vi "Teleop.vi"(10 "Match Info":T13={"Autonomous Elapsed Seconds"=0.0, "TeleOp Elapsed Seconds"=0.0, "Disabled Elapsed Seconds"=0.0, "Visited Autonomous"=FALSE, "Visited TeleOp"=FALSE, "Visited Disabled"=FALSE, "Autonomous Settings"={"Autonomous Style"=enum."Independent", "VI Refnum"=refnum}}, 11 "Call Context":T14) -> ()   [LabVIEW 2014]
doc: "This VI is called for each TeleOp packet received from the DS where the robot is not disabled. It is often used to read from the joysticks and update I/O or to update setpoints for timed control loops. It should complete and return within 20 milliseconds or it may miss DS packets."
uses:
  <vilib>/Rock Robotics/WPI/DriverStation/WPI_DriverStationDerivedRobotMode.ctl
  <vilib>/Rock Robotics/WPI/DriverStation/WPI_DriverStationMatch Info.ctl
  <vilib>/Rock Robotics/WPI/Joystick/WPI_JoystickDevRef.ctl
  <vilib>/Rock Robotics/WPI/Joystick/WPI_JoystickDeviceEnum.ctl
  <vilib>/Rock Robotics/WPI/RobotDrive/WPI_RobotDriveDevRef.ctl
  <vilib>/Rock Robotics/WPI/MotorControl/WPI_MotorControlDeviceRef.ctl
  <vilib>/Rock Robotics/WPI/MotorControl/WPI_MotorControlType.ctl
  <vilib>/Rock Robotics/SystemInterfaces/Typedef/FPGA_TypedefDigitalModule.ctl
  <vilib>/Rock Robotics/SystemInterfaces/DIO/FPGA_DIOPWMChannel.ctl
  <vilib>/Rock Robotics/WPI/PWM/WPI_PWMDeadband.ctl
  <vilib>/Rock Robotics/WPI/CAN/Jaguar/SubVIs/WPI_CANJaguar_ControlMode.ctl
  <vilib>/Rock Robotics/WPI/CAN/TalonSRX/WPI_CANTalonSRX_APIControlMode.ctl
  <vilib>/Rock Robotics/WPI/PWM/WPI_PWMTransform_ConPane.ctl
  <vilib>/Rock Robotics/WPI/Solenoid/WPI_SolenoidValue.ctl
  <vilib>/Rock Robotics/Network Tables/SD Read Boolean.vi
  <vilib>/Rock Robotics/Network Tables/SD Read Number.vi
  <vilib>/Rock Robotics/WPI/Joystick/WPI_JoystickGetSetRefNum.vi
  <vilib>/Rock Robotics/Network Tables/SD Read Boolean Array.vi
  <vilib>/Rock Robotics/WPI/RobotDrive/WPI_RobotDriveGetSetRefNum.vi
  <vilib>/Rock Robotics/Network Tables/SD Write Numeric Array.vi
  Robot Global Data.vi
  <vilib>/Rock Robotics/WPI/Solenoid/WPI_SolenoidSetEnum.vi
  <vilib>/Rock Robotics/Network Tables/SD Write Boolean Array.vi
  <vilib>/Rock Robotics/WPI/RobotDrive/WPI_RobotDriveMecanumDrive_Cartesian.vi
panel:
  out "Mecanum_Motors":T1={"DevStatus"={"status"=FALSE, "code"=0, "source"=""}, "Motors[]"=[], "Square Inputs"=FALSE, "Max Output"=1.0}
  out "Numeric":dbl
  out "Boolean Array":bool[](array[boolean])
  in  "Radio Buttons":enum32{"Radio Selection 1", "Radio Selection 2"}(radio)
  out "Joystick_1":T11={"Device"=enum."USB 1"}
  out "Joystick_0":T11={"Device"=enum."USB 1"}
  out "Sample Slider 0":dbl(slide) scale=0.0..5.0
  out "Sample Boolean 1":bool
  out "Sample Boolean 0":bool
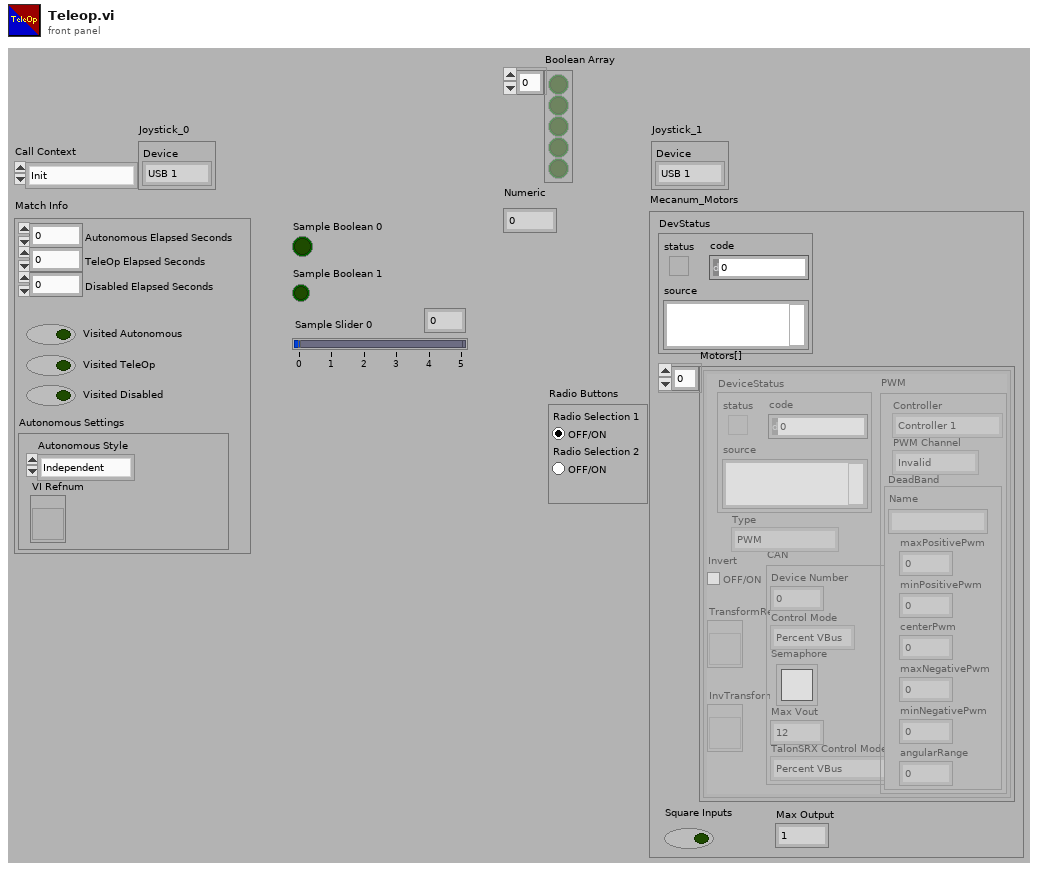
[diagram p1: front panel]
types:
  T1 = typedef "WPI_RobotDriveDevRef.ctl" = cluster{"DevStatus":errorcluster, "Motors[]":T2[], "Square Inputs":bool, "Max Output":dbl}
  T2 = typedef "WPI_MotorControlDeviceRef.ctl" = cluster{"DeviceStatus":errorcluster, "Type":T3, "PWM":cluster{"Controller":T4, "PWM Channel":T5, "DeadBand":T6}, "CAN":cluster{"Device Number":u8, "Control Mode":T7, "Semaphore":T8, "Max Vout":dbl, "TalonSRX Control Mode":T9}, "Invert":bool, "TransformRef":T10, "InvTransformRef":T10}
  T3 = typedef "WPI_MotorControlType.ctl" = enum16{"PWM", "CAN", "CANTalonSRX"}
  T4 = typedef "FPGA_TypedefDigitalModule.ctl" = enum16{"Controller 1"}
  T5 = typedef "FPGA_DIOPWMChannel.ctl" = enum8{"PWM 0", "PWM 1", "PWM 2", "PWM 3", "PWM 4", "PWM 5", "PWM 6", "PWM 7", "PWM 8", "PWM 9", "PWM MXP 0", "PWM MXP 1", "PWM MXP 2", "PWM MXP 3", "PWM MXP 4", "PWM MXP 5", "PWM MXP 6", "PWM MXP 7", "PWM MXP 8", "PWM MXP 9", "Invalid"}
  T6 = typedef "WPI_PWMDeadband.ctl" = cluster{"Name":string, "maxPositivePwm":i32, "minPositivePwm":i32, "centerPwm":i32, "maxNegativePwm":i32, "minNegativePwm":i32, "angularRange":u16}
  T7 = typedef "WPI_CANJaguar_ControlMode.ctl" = enum8{"Percent VBus", "Current", "Speed", "Position", "Voltage"}
  T8 = typedef "Semaphore RefNum" = refnum<k1>
  T9 = typedef "WPI_CANTalonSRX_APIControlMode.ctl" = enum8{"Percent VBus", "Speed", "Position", "Slave", "Unchanged / Invalid"}
  T10 = typedef "WPI_PWMTransform_ConPane.ctl" = refnum<vi>
  T11 = typedef "WPI_JoystickDevRef.ctl" = cluster{"Device":T12}
  T12 = typedef "WPI_JoystickDeviceEnum.ctl" = enum16{"USB 0", "USB 1", "USB 2", "USB 3", "USB 4", "USB 5"}
  T13 = typedef "WPI_DriverStationMatch Info.ctl" = cluster{"Autonomous Elapsed Seconds":dbl, "TeleOp Elapsed Seconds":dbl, "Disabled Elapsed Seconds":dbl, "Visited Autonomous":bool, "Visited TeleOp":bool, "Visited Disabled":bool, "Autonomous Settings":cluster{"Autonomous Style":enum16{"Iterative", "Independent"}, "VI Refnum":refnum<vi>}}
  T14 = typedef "WPI_DriverStationDerivedRobotMode.ctl" = enum16{"Init", "Execute", "Stop"}
  T15 = typedef "WPI_SolenoidValue.ctl" = enum16{"Off", "On", "Forward", "Reverse"}
  T16 = typedef "WPI_SolenoidDevRef.ctl" = cluster{"DevStatus":errorcluster, "Pneumatics Control Module":u8, "Forward Solenoid Channel":T17, "Reverse Solenoid Channel":T17}
  T17 = typedef "WPI_SolenoidChannel.ctl" = enum8{"Solenoid 0", "Solenoid 1", "Solenoid 2", "Solenoid 3", "Solenoid 4", "Solenoid 5", "Solenoid 6", "Solenoid 7", "Invalid"}
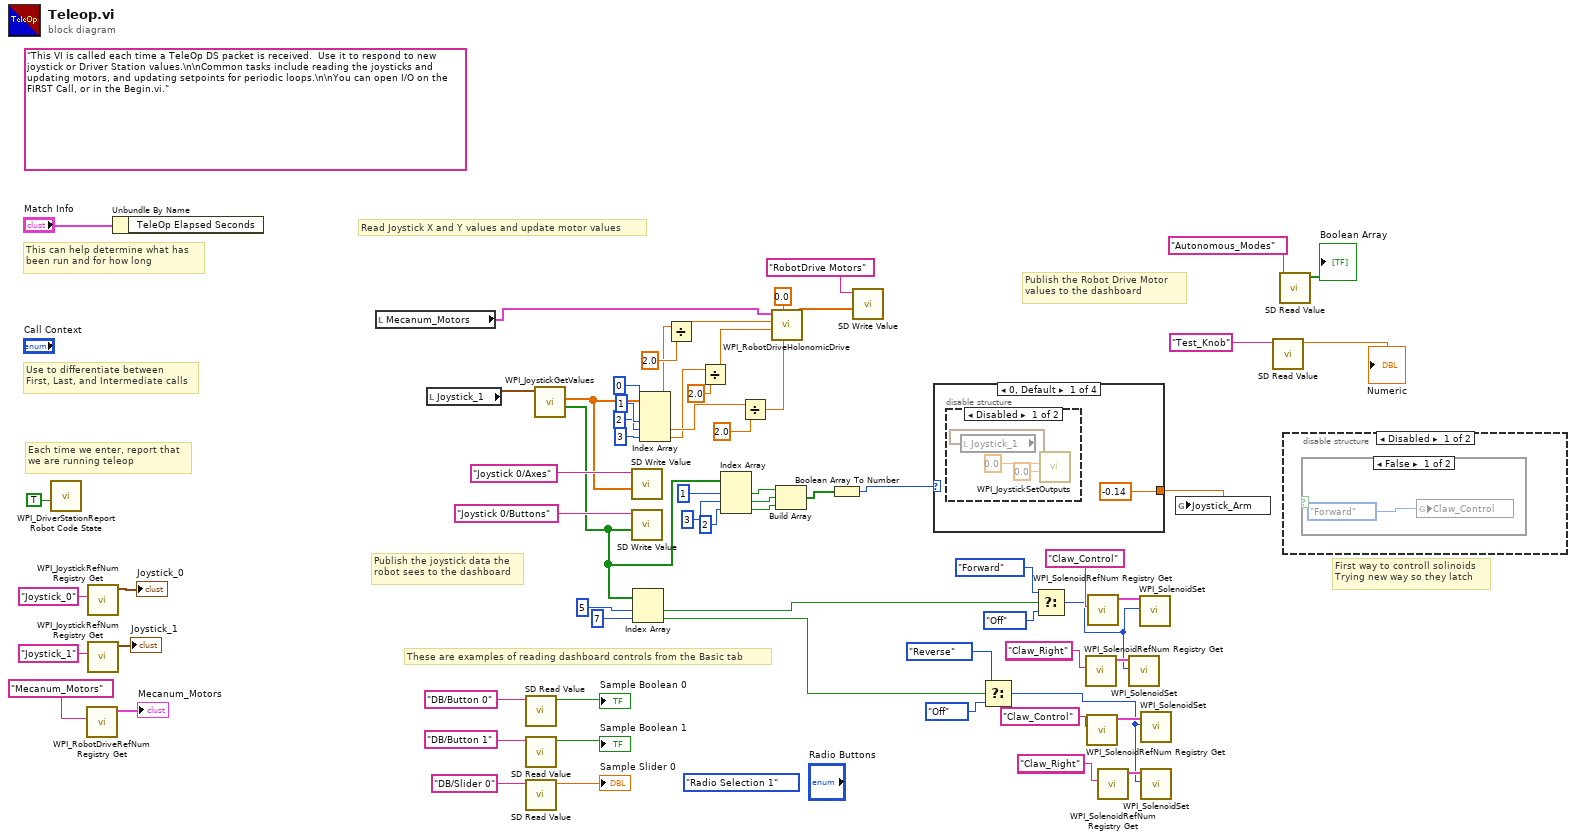
[diagram p0: block diagram]
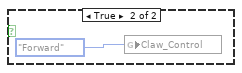
[diagram p2: hidden frame]
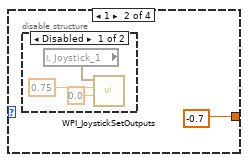
[diagram p5: hidden frame]
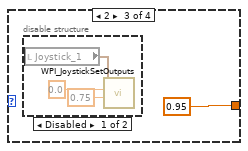
[diagram p7: hidden frame]
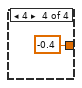
[diagram p9: hidden frame]
diagram:
  (unwired) "Claw_Right" ("refnum name")
  (unwired) "Claw_Right" ("refnum name")
  (unwired) enum32{"Radio Selection 1", "Radio Selection 2"}."Radio Selection 1" ("Radio Buttons")
  (unwired) "This VI is called each time a TeleOp DS packet is received.  Use it to respond to new joystick or Driver Station values.\n\nCommon tasks include reading the joysticks and updating motors, and updating setpoints for periodic loops.\n\nYou can open I/O on the FIRST Call, or in the Begin.vi."
  # "First way to controll solinoids\nTrying new way so they latch"
  # "These are examples of reading dashboard controls from the Basic tab"
  # "Publish the Robot Drive Motor\nvalues to the dashboard"
  # "Publish the joystick data the\nrobot sees to the dashboard"
  # "Each time we enter, report that\nwe are running teleop"
  # "Use to differentiate between\nFirst, Last, and Intermediate calls"
  # "This can help determine what has\nbeen run and for how long"
  # "Read Joystick X and Y values and update motor values"
  n1 = call <vilib>:"WPI_DriverStationReport Robot Code State.vi"("TeleOp"=TRUE ("Autonomous")) -> ()  [unwired: 10 in, 1 out]
  n2 = call <vilib>:"WPI_RobotDriveRefNum Registry Get.vi"("refnum name"="Mecanum_Motors") -> ("RobotDriveDevRef"=→"Mecanum_Motors":T1)  [unwired: 1 in, 9 out]
  n3 = call <vilib>:"WPI_JoystickRefNum Registry Get.vi"("refnum name"="Joystick_0") -> ("JoystickDevRef"=→"Joystick_0":T11)  [unwired: 9 in, 1 out]
  n4 = call <vilib>:"WPI_JoystickRefNum Registry Get.vi"("refnum name"="Joystick_1") -> ("JoystickDevRef"=→"Joystick_1":T11)  [unwired: 9 in, 1 out]
  n5 = Unbundle By Name("Match Info") -> ()  [unwired: 1 out]
  n6 = local read "Mecanum_Motors"() -> (w36:T1)
  n7 = local read "Joystick_1"() -> (w39:T11)
  n8 = call-poly <vilib>:"SD Read Value.vi"("Name"="DB/Button 0" ("refnum name")) -> ("Boolean"=→"Sample Boolean 0":bool)  [unwired: 8 in, 2 out]
  n9 = call-poly <vilib>:"SD Read Value.vi"("Name"="DB/Button 1" ("refnum name")) -> ("Boolean"=→"Sample Boolean 1":bool)  [unwired: 8 in, 2 out]
  n10 = call-poly <vilib>:"SD Read Value.vi"("Name"="DB/Slider 0" ("refnum name")) -> ("Numeric"=→"Sample Slider 0":dbl)  [unwired: 8 in, 2 out]
  n11 = call <vilib>:"WPI_JoystickGetValues.vi"("JoystickDevRef"=w39) -> ("Buttons"=w35:bool[], "Axes"=w51:dbl[])  [unwired: 6 in, 3 out]
  n12 = call-poly <vilib>:"SD Write Value.vi"("Numeric Array"=w51, "Name"="Joystick 0/Axes") -> ()  [unwired: 8 in, 2 out]
  n13 = call-poly <vilib>:"SD Write Value.vi"("Boolean Array"=w35, "Name"="Joystick 0/Buttons") -> ()  [unwired: 8 in, 2 out]
  n14 = Index Array(array=w35, index #1=5 ("index"), index #2=7 ("index")) -> (element #1=w27:bool, element #2=w16:bool)
  n15 = Index Array(array=w51, index #1=0, index #2=1, index #3=2 ("index"), index #4=3 ("index")) -> (element #1=w8:dbl, element #3=w13:dbl, element #4=w10:dbl)  [unwired: 1 out]
  n16 = Divide(x=w8, y=2.0) -> (x/y=w7:dbl)
  n17 = Divide(x=w10, y=2.0) -> (x/y=w9:dbl)
  n18 = Index Array(array=w35, index #1=1, index #2=3, index #3=2 ("index")) -> (element #1=w32:bool, element #2=w31:bool, element #3=w17:bool)
  n19 = Divide(x=w13, y=2.0) -> (x/y=w15:dbl)
  n20 = call-poly <vilib>:"WPI_RobotDriveHolonomicDrive.vi"("Rotation"=w15, "Gyro Angle"=0.0, "Y"=w9, "X"=w7, "RobotDriveDevRef"=w36) -> ("Motor Values"=w58:dbl[])  [unwired: 4 in, 2 out]
  n21 = Build Array(w32, w31, w17) -> (w30:bool[])
  n22 = Boolean Array To Number(Boolean array=w30) -> (number=w29:u32)
  n23 = call-poly <vilib>:"SD Write Value.vi"("Numeric Array"=w58, "Name"="RobotDrive Motors") -> ()  [unwired: 8 in, 2 out]
  n24 = case shown="0, Default" w29 {
    tunnel: [-0.14 -0.7 0.95 -0.4] -> w48
    frame 0, Default {
      n25 = disable-structure shown="Disabled" {
        frame Disabled {
          n26 = local read "Joystick_1"() -> (w69:T11)
          n27 = call <vilib>:"WPI_JoystickSetOutputs.vi"("Right Rumble"=sgl 0.0, "Left Rumble"=sgl 0.0, "JoystickDevRef"=w69) -> ()  [unwired: 7 in, 2 out]
        }
        frame Enabled {
        }
      }
    }
    frame 1 {
      n28 = disable-structure shown="Disabled" {
        frame Disabled {
          n29 = local read "Joystick_1"() -> (w75:T11)
          n30 = call <vilib>:"WPI_JoystickSetOutputs.vi"("Right Rumble"=sgl 0.0, "Left Rumble"=sgl 0.75, "JoystickDevRef"=w75) -> ()  [unwired: 7 in, 2 out]
        }
        frame Enabled {
        }
      }
    }
    frame 2 {
      n31 = disable-structure shown="Disabled" {
        frame Disabled {
          n32 = local read "Joystick_1"() -> (w77:T11)
          n33 = call <vilib>:"WPI_JoystickSetOutputs.vi"("Right Rumble"=sgl 0.75, "Left Rumble"=sgl 0.0, "JoystickDevRef"=w77) -> ()  [unwired: 7 in, 2 out]
        }
        frame Enabled {
        }
      }
    }
    frame 4 {
    }
  }
  n34 = Select(t=WPI_SolenoidValue."Reverse" ("Claw_Control"), s=w16, f=WPI_SolenoidValue."Off" ("Claw_Control")) -> (s? t:f=w1:T15)
  n35 = Select(t=WPI_SolenoidValue."Forward" ("Claw_Control"), s=w27, f=WPI_SolenoidValue."Off" ("Claw_Control")) -> (s? t:f=w4:T15)
  n36 = call <vilib>:"WPI_SolenoidRefNum Registry Get.vi"("refnum name"="Claw_Right") -> ("SolenoidDevRef"=w6:T16)  [unwired: 9 in, 1 out]
  n37 = call <vilib>:"WPI_SolenoidRefNum Registry Get.vi"("refnum name"="Claw_Control") -> ("SolenoidDevRef"=w22:T16)  [unwired: 9 in, 1 out]
  n38 = call <vilib>:"WPI_SolenoidRefNum Registry Get.vi"("refnum name"="Claw_Control") -> ("SolenoidDevRef"=w21:T16)  [unwired: 9 in, 1 out]
  n39 = call <vilib>:"WPI_SolenoidRefNum Registry Get.vi"("refnum name"="Claw_Right") -> ("SolenoidDevRef"=w2:T16)  [unwired: 9 in, 1 out]
  n40 = call-poly <vilib>:"WPI_SolenoidSet.vi"("Value"=w4, "SolenoidDevRef"=w6) -> ()  [unwired: 8 in, 2 out]
  n41 = call-poly <vilib>:"WPI_SolenoidSet.vi"("Value"=w4, "SolenoidDevRef"=w21) -> ()  [unwired: 8 in, 2 out]
  n42 = call-poly <vilib>:"WPI_SolenoidSet.vi"("Value"=w1, "SolenoidDevRef"=w22) -> ()  [unwired: 8 in, 2 out]
  n43 = call-poly <vilib>:"WPI_SolenoidSet.vi"("Value"=w1, "SolenoidDevRef"=w2) -> ()  [unwired: 8 in, 2 out]
  n44 = global write "Robot Global Data.vi" "Joystick_Arm"(w48) -> ()
  n45 = call-poly <vilib>:"SD Read Value.vi"("Name"="Test_Knob") -> ("Numeric"=→"Numeric":dbl)  [unwired: 8 in, 2 out]
  n46 = call-poly <vilib>:"SD Read Value.vi"("Name"="Autonomous_Modes") -> ("Boolean Array"=→"Boolean Array":bool[])  [unwired: 8 in, 2 out]
  n47 = disable-structure shown="Disabled" {
    frame Disabled {
      n48 = case shown="False" {
        selector: _ -> [_ _]
        frame False {
          n49 = global write "Robot Global Data.vi" "Claw_Control"(WPI_SolenoidValue."Forward" ("Claw_Control")) -> ()
        }
        frame True {
          n50 = global write "Robot Global Data.vi" "Claw_Control"(WPI_SolenoidValue."Forward" ("Claw_Control")) -> ()
        }
      }
    }
    frame Enabled {
    }
  }
